vi "data sorting to sequence 17O Simple.vi"(8 "error in":errorcluster) -> (3 "cycle results cluster out":T1, 11 "cycle results cluster IN":T1)   [LabVIEW 2016]
doc: "Takes a sample type and sorts by sequence"
uses:
  controls/cycle results control.ctl
  controls/data control cluster.ctl
  <vilib>/Analysis/baseanly.llb/Mean (DBL).vi
  <vilib>/Analysis/NI_AALBase.lvlib
panel:
  out "error out":errorcluster
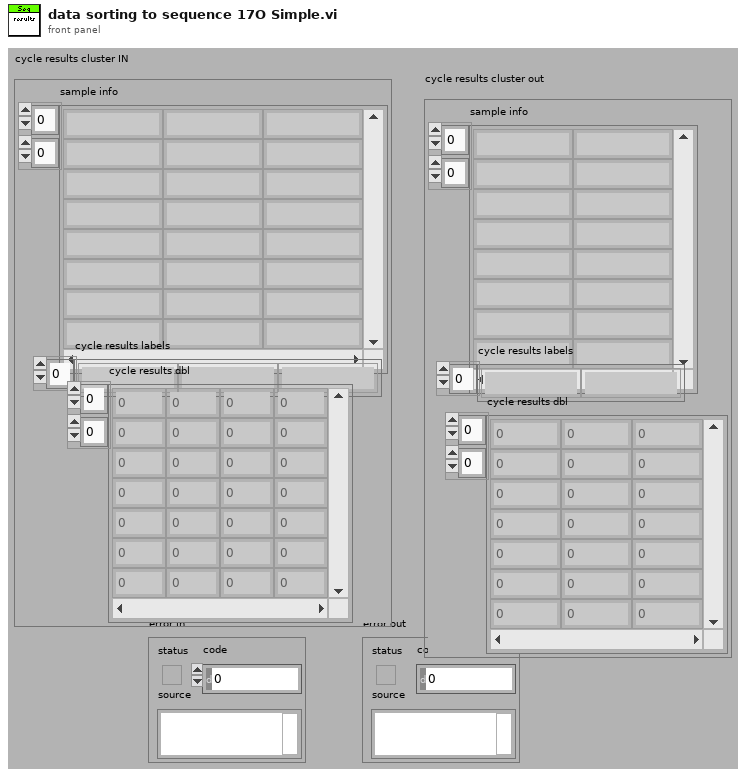
[diagram p1: front panel]
types:
  T1 = typedef "cycle results control.ctl" = cluster{"sample info":string[][], "cycle results labels":string[], "cycle results dbl":dbl[][]}
  T2 = typedef "data control cluster.ctl" = cluster{"Final result header":string[], "sequence result header":string[], "cycle result header ":string[], "Final Result":string[][], "sequence  Result":dbl[][], "Cycle data by seq":dbl[][][], "Cycle data by position":dbl[][][], "Final seq  Result":dbl[][], "only specific type":dbl[][]}
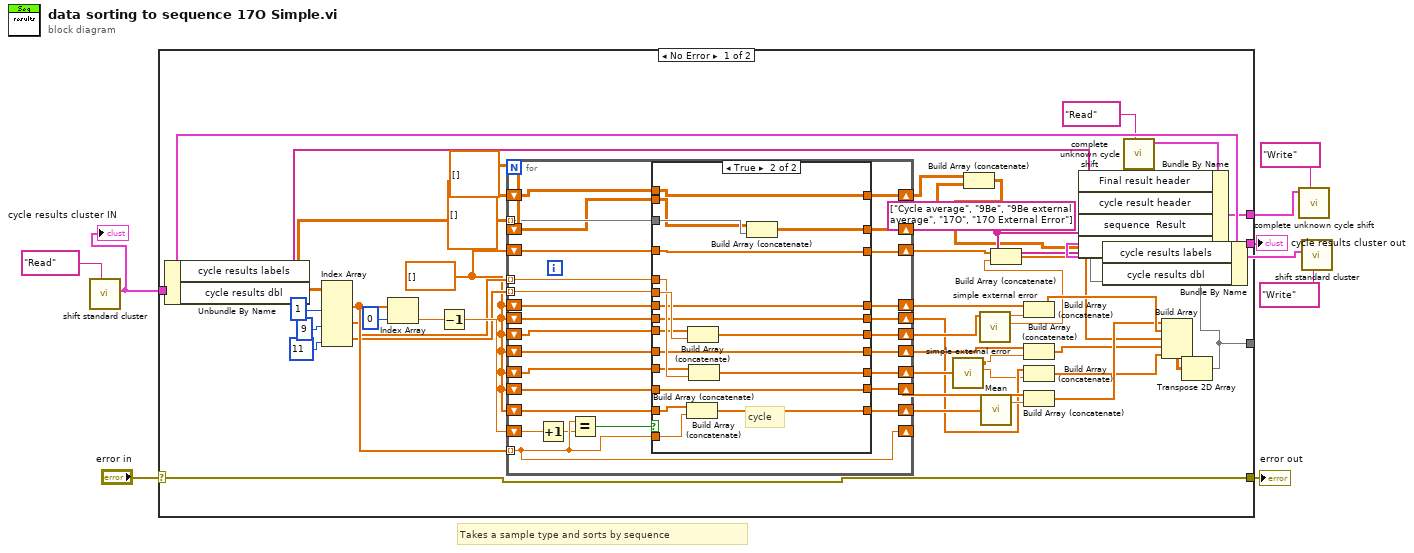
[diagram p0: block diagram]
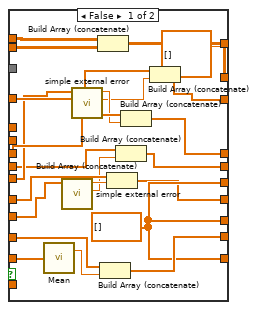
[diagram p2: hidden frame]
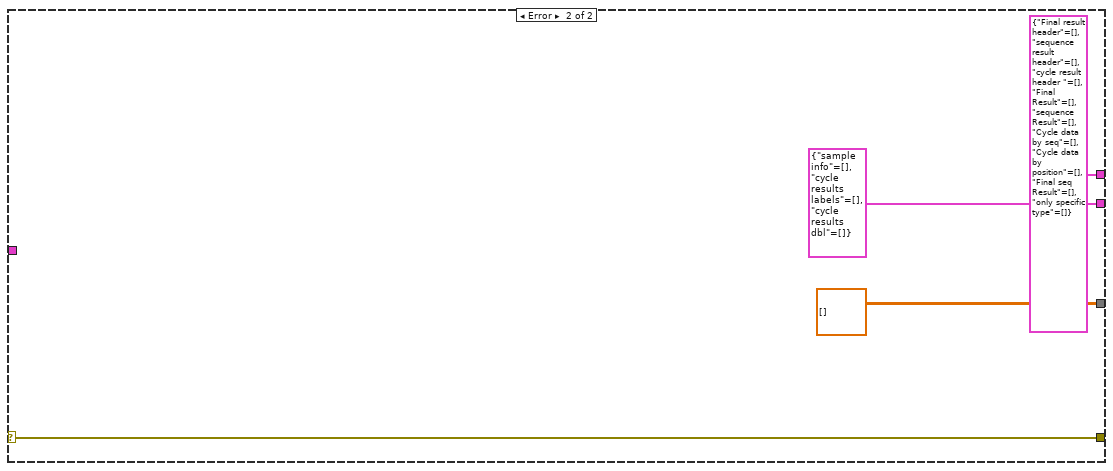
[diagram p3: hidden frame]
diagram:
  # "Takes a sample type and sorts by sequence"
  n1 = call "shift standard cluster.vi"("read write shift"="Read") -> ("cycle results cluster out"=w3:T1)  [unwired: 9 in, 1 out]
  "cycle results cluster IN" <- w3
  n2 = case shown="No Error" "error in" {
    selector: "error in" -> [w36 w123]
    tunnel: w3 -> [w35 _]
    tunnel: [w11 dbl[][] []] -> _
    tunnel: [w34 T1 {"sample info"=[], "cycle results labels"=[], "cycle results dbl"=[]} ("cycle results cluster IN")] -> w5
    tunnel: [w36 w123] -> w7
    tunnel: [w10 T2 {"Final result header"=[], "sequence result header"=[], "cycle result header "=[], "Final Result"=[], "sequence  Result"=[], "Cycle data by seq"=[], "Cycle data by position"=[], "Final seq  Result"=[], "only specific type"=[]} ("DATA CLUSTER out")] -> w1
    frame No Error {
      w13 = string[] ["Cycle average", "9Be", "9Be external average", "17O", "17O External Error"] ("cycle results labels")
      w21 = dbl[] []
      n3 = Unbundle By Name(w35) -> ("cycle results labels"=w9:string[], "cycle results dbl"=w20:dbl[][])
      n4 = Index Array(array=w20, index (col) #1=1 ("disabled index (col)"), index (col) #2=9 ("index (col)"), index (col) #3=11 ("index (col)")) -> (element #1=w41:dbl[], element #2=w40:dbl[], element #3=w39:dbl[])  [unwired: 3 in]
      n5 = Index Array(array=w41, index=0) -> (element=w47:dbl)
      n6 = Decrement(x=w47) -> (x-1=w46:dbl)
      n7 = for {
        tunnel: w41 -> [w73] mode=indexing
        shift-right: [w77] -> w48
        shift-left: w21 -> [w76]
        shift-right: [w75] -> w52
        shift-left: w21 -> [w74]
        shift-right: [w73] -> _
        shift-left: w46 -> [w79]
        tunnel: w39 -> [w72] mode=indexing
        tunnel: w40 -> [w71] mode=indexing
        shift-right: [w70] -> w28
        shift-left: w21 -> [w67]
        shift-right: [w69] -> w32
        shift-left: w21 -> [w68]
        shift-right: [w66] -> w49
        shift-left: w21 -> [w64]
        shift-right: [w65] -> w50
        shift-left: w21 -> [w63]
        shift-right: [w61] -> w29
        shift-left: w21 -> [w60]
        shift-right: [w59] -> w26
        shift-left: w21 -> [w58]
        tunnel: w20 -> [w57] mode=indexing
        shift-right: [w56] -> w16
        shift-left: dbl[][] [] -> [w55]
        shift-right: [w54] -> w17
        shift-left: dbl[][][] [] -> [w53]
        n8 = Increment(x=w79) -> (x+1=w62:dbl)
        n9 = Equal?(x=w73, y=w62) -> (x = y?=w78:bool)
        n10 = case shown="True" w78 {
          tunnel: w73 -> [_ w117]
          tunnel: [w98 w120] -> w77
          tunnel: w76 -> [w102 w118]
          tunnel: [w101 w119] -> w75
          tunnel: w74 -> [w100 w119]
          tunnel: w72 -> [_ w116]
          tunnel: w71 -> [_ w115]
          tunnel: [w98 w114] -> w70
          tunnel: [w98 w113] -> w69
          tunnel: w68 -> [w90 w112]
          tunnel: w67 -> [w88 w111]
          tunnel: [w97 w110] -> w66
          tunnel: [w96 w109] -> w65
          tunnel: w64 -> [w95 w110]
          tunnel: w63 -> [w94 w109]
          tunnel: [w93 w108] -> w61
          tunnel: w60 -> [w92 w108]
          tunnel: [w85 w107] -> w59
          tunnel: w58 -> [w84 w107]
          tunnel: w57 -> [_ w106]
          tunnel: [dbl[][] [] w105] -> w56
          tunnel: w55 -> [w83 w103]
          tunnel: [w82 w104] -> w54
          tunnel: w53 -> [w81 w104]
          frame False {
            w98 = dbl[] []
            n11 = call-poly <vilib>:"Mean.vi"("X"=w102) -> ("mean"=w99:dbl)  [unwired: 1 out]
            n12 = call "simple external error.vi"("cycle results"=w88) -> ("External error"=w86:dbl, "Sequence result"=w87:dbl)  [unwired: 7 in, 2 out]
            n13 = call "simple external error.vi"("cycle results"=w90) -> ("External error"=w89:dbl, "Sequence result"=w91:dbl)  [unwired: 7 in, 2 out]
            n14 = Build Array (concatenate)(w81, w83) -> (w82:dbl[][][])
            n15 = Build Array (concatenate)(w100, w99) -> (w101:dbl[])
            n16 = Build Array (concatenate)(w94, w87) -> (w96:dbl[])
            n17 = Build Array (concatenate)(w84, w86) -> (w85:dbl[])
            n18 = Build Array (concatenate)(w95, w91) -> (w97:dbl[])
            n19 = Build Array (concatenate)(w92, w89) -> (w93:dbl[])
          }
          frame True {
            # "cycle"
            n20 = Build Array (concatenate)(w118, w117) -> (w120:dbl[])
            n21 = Build Array (concatenate)(w112, w116) -> (w113:dbl[])
            n22 = Build Array (concatenate)(w111, w115) -> (w114:dbl[])
            n23 = Build Array (concatenate)(w103, w106) -> (w105:dbl[][])
          }
        }
      }
      n24 = call "simple external error.vi"("cycle results"=w28) -> ("External error"=w25:dbl, "Sequence result"=w27:dbl)  [unwired: 7 in, 2 out]
      n25 = Build Array (concatenate)(w17, w16) -> (w12:dbl[][][])
      n26 = call "simple external error.vi"("cycle results"=w32) -> ("External error"=w30:dbl, "Sequence result"=w31:dbl)  [unwired: 7 in, 2 out]
      n27 = call-poly <vilib>:"Mean.vi"("X"=w48) -> ("mean"=w51:dbl)  [unwired: 1 out]
      n28 = Build Array (concatenate)(w29, w30) -> (w24:dbl[])
      n29 = Build Array (concatenate)(w49, w31) -> (w38:dbl[])
      n30 = Build Array (concatenate)(w50, w27) -> (w23:dbl[])
      n31 = Build Array (concatenate)(w26, w25) -> (w22:dbl[])
      n32 = Build Array (concatenate)(w52, w51) -> (w37:dbl[])
      n33 = call "complete unknown cycle shift.vi"("read write shift"="Read") -> ("DATA CLUSTER out"=w15:T2)  [unwired: 9 in, 1 out]
      n34 = Build Array(w37, w38, w24, w23, w22) -> (w33:dbl[][])
      n35 = Transpose 2D Array(2D array=w33) -> (transposed array=w11:dbl[][])
      n36 = Bundle By Name(cluster=w15, "Final result header"=w13, "cycle result header"=w9, "sequence  Result"=w11, "Cycle data by seq"=w12) -> (w10:T2)
      n37 = Bundle By Name(cluster=w35, "cycle results labels"=w13, "cycle results dbl"=w11) -> (w34:T1)
    }
    frame Error {
    }
  }
  "error out" <- w7
  "cycle results cluster out" <- w5
  n38 = call "complete unknown cycle shift.vi"("read write shift"="Write", "DATA CLUSTER in"=w1) -> ()  [unwired: 8 in, 2 out]
  n39 = call "shift standard cluster.vi"("read write shift"="Write", "cycle results cluster In"=w5) -> ()  [unwired: 8 in, 2 out]
